vi "FilterWheelSub.vi"(2 "TFW Serial Port":string="COM17") -> ()   [LabVIEW 2018]
doc: "This example shows how to acquire a power measurement using the VIs of the driver."
uses:
  Global Variables.vi
  <vilib>/Utility/file.llb/Read Delimited Spreadsheet (string).vi
  <instrlib>/Thorlabs_FW102C/Thorlabs_FW102C.lvlib
panel:
  out "Position Error?":bool
  out "Position Error?":bool
  in  "stop":bool
  in  "RFW Serial Port":string="COM17"
  out "RFW102C out":i32
  in  "RFW Wavelengths":u16(ring) items=["800", "900", "850", "750", "700", "600"]
  out "RFW wls":dbl[](array[numeric])
  out "TFW wls":dbl[](array[numeric])
  in  "TFW Wavelengths":u16(ring) items=["1000", "850", "800", "700", "650", "600"]
  out "error out":errorcluster
  out "TFW102C out":i32
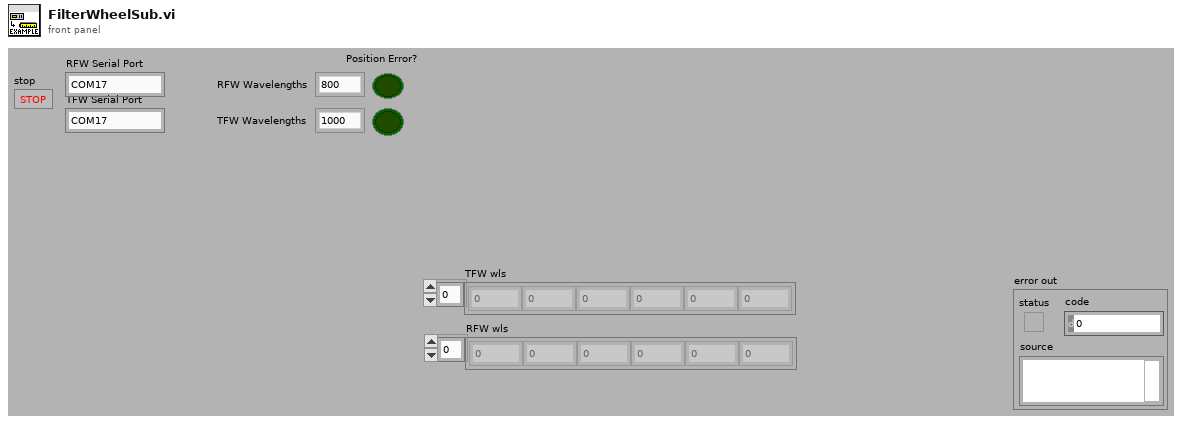
[diagram p1: front panel]
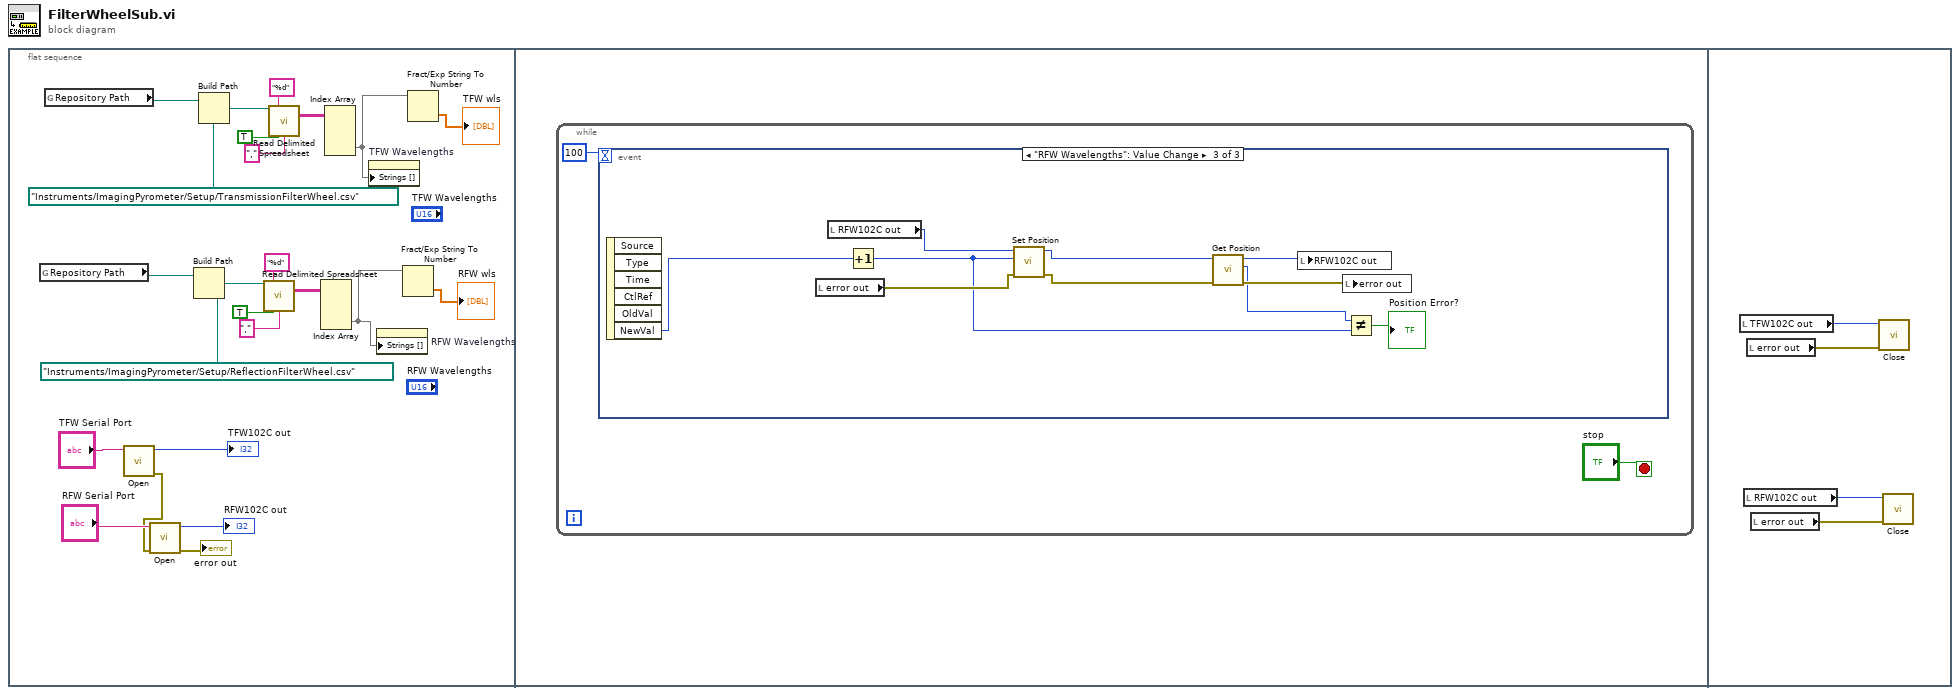
[diagram p0: block diagram]
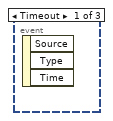
[diagram p2: hidden frame]
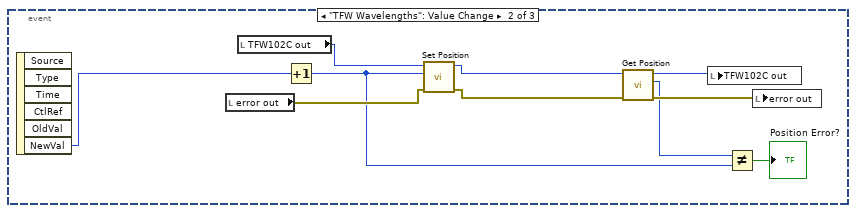
[diagram p3: hidden frame]
diagram:
  n1 = flat-sequence {
    frame #0 {
      n2 = global read "Global Variables.vi" "Repository Path"() -> (w9:path)
      n3 = global read "Global Variables.vi" "Repository Path"() -> (w18:path)
      n4 = call <instrlib>:"Open.vi"("Serial Port"="TFW Serial Port") -> ("error out"=w2:errorcluster, "FW102C out"=→"TFW102C out":i32)  [unwired: 8 in, 1 out]
      n5 = call <instrlib>:"Open.vi"("error in (no error)"=w2, "Serial Port"="RFW Serial Port") -> ("error out"=→"error out":errorcluster, "FW102C out"=→"RFW102C out":i32)  [unwired: 7 in, 1 out]
      n6 = Build Path(base path=w9, name or relative path=path "Instruments/ImagingPyrometer/Setup/ReflectionFilterWheel.csv" ("vi path")) -> (appended path=w8:path)
      n7 = Build Path(base path=w18, name or relative path=path "Instruments/ImagingPyrometer/Setup/TransmissionFilterWheel.csv" ("vi path")) -> (appended path=w19:path)
      n8 = call-poly <vilib>:"Read Delimited Spreadsheet.vi"("file path (dialog if empty)"=w8, "format (%s)"="%d", "transpose? (F)"=TRUE, "delimiter (\\t)"="," ("delimiter (\\t)")) -> ("all rows"=w11:string[][])  [unwired: 6 in, 5 out]
      n9 = call-poly <vilib>:"Read Delimited Spreadsheet.vi"("file path (dialog if empty)"=w19, "format (%s)"="%d", "transpose? (F)"=TRUE, "delimiter (\\t)"="," ("delimiter (\\t)")) -> ("all rows"=w16:string[][])  [unwired: 6 in, 5 out]
      n10 = Index Array(array=w11) -> (element #2=w13:string[])  [unwired: 4 in, 1 out]
      n11 = Index Array(array=w16) -> (element #2=w14:string[])  [unwired: 4 in, 1 out]
      n12 = property on="TFW Wavelengths" class="Ring (strict)"("Strings []"=w14) -> ()  [unwired: 2 in, 2 out]
      n13 = property on="RFW Wavelengths" class="Ring (strict)"("Strings []"=w13) -> ()  [unwired: 2 in, 2 out]
      n14 = Fract/Exp String To Number(string=w13) -> (number=→"RFW wls":dbl[])  [unwired: 3 in, 1 out]
      n15 = Fract/Exp String To Number(string=w14) -> (number=→"TFW wls":dbl[])  [unwired: 3 in, 1 out]
    }
    frame #1 {
      n16 = while {
        stop <- "stop" stop-if-true
        n17 = event shown="[2] \"RFW Wavelengths\": Value Change" {
          selector: _ -> [_ _ _]
          dyn-events: _ -> [_ _ _]
          timeout: u32 100 ("milliseconds to wait") -> [_ _ _]
          event Timeout {
            n18 = event-data() -> ()  [unwired: 1 in, 3 out]
          }
          event "TFW Wavelengths": Value Change {
            n19 = event-data() -> ("NewVal"=w30:u16)  [unwired: 1 in, 5 out]
            n20 = local read "error out"() -> (w35:errorcluster)
            n21 = local read "TFW102C out"() -> (w36:i32)
            n22 = Increment(x=w30) -> (x+1=w28:u16)
            n23 = call <instrlib>:"Set Position.vi"("error in (no error)"=w35, "Position"=w28, "FW102C in"=w36) -> ("error out"=w33:errorcluster, "FW102C out"=w34:i32)  [unwired: 7 in]
            n24 = call <instrlib>:"Get Position.vi"("error in (no error)"=w33, "FW102C in"=w34) -> ("error out"=w31:errorcluster, "Position"=w29:i32, "FW102C out"=w32:i32)  [unwired: 7 in]
            n25 = local write "TFW102C out"(w32) -> ()
            n26 = Not Equal?(x=w29, y=w28) -> (x != y?=→"Position Error?":bool)
            n27 = local write "error out"(w31) -> ()
          }
          event "RFW Wavelengths": Value Change {
            n28 = event-data() -> ("NewVal"=w40:u16)  [unwired: 1 in, 5 out]
            n29 = local read "error out"() -> (w45:errorcluster)
            n30 = local read "RFW102C out"() -> (w46:i32)
            n31 = Increment(x=w40) -> (x+1=w39:u16)
            n32 = call <instrlib>:"Set Position.vi"("error in (no error)"=w45, "Position"=w39, "FW102C in"=w46) -> ("error out"=w43:errorcluster, "FW102C out"=w44:i32)  [unwired: 7 in]
            n33 = call <instrlib>:"Get Position.vi"("error in (no error)"=w43, "FW102C in"=w44) -> ("error out"=w41:errorcluster, "Position"=w38:i32, "FW102C out"=w42:i32)  [unwired: 7 in]
            n34 = local write "RFW102C out"(w42) -> ()
            n35 = local write "error out"(w41) -> ()
            n36 = Not Equal?(x=w38, y=w39) -> (x != y?=→"Position Error?":bool)
          }
        }
      }
    }
    frame #2 {
      n37 = local read "TFW102C out"() -> (w49:i32)
      n38 = local read "RFW102C out"() -> (w48:i32)
      n39 = local read "error out"() -> (w50:errorcluster)
      n40 = local read "error out"() -> (w47:errorcluster)
      n41 = call <instrlib>:"Close.vi"("error in (no error)"=w50, "FW102C in"=w49) -> ()  [unwired: 9 in, 1 out]
      n42 = call <instrlib>:"Close.vi"("error in (no error)"=w47, "FW102C in"=w48) -> ()  [unwired: 9 in, 1 out]
    }
  }
